vi "FindSimETH_CAn.vi"(6 "COM":string, 8 "error in":errorcluster) -> (0 "error out":errorcluster, 1 "Pass":bool, 2 "CmdOut":string)   [LabVIEW 2013]
panel:
  out "连接的字符串":string
  out "x >= 0?":bool
  out "数组":string[][](array[string])
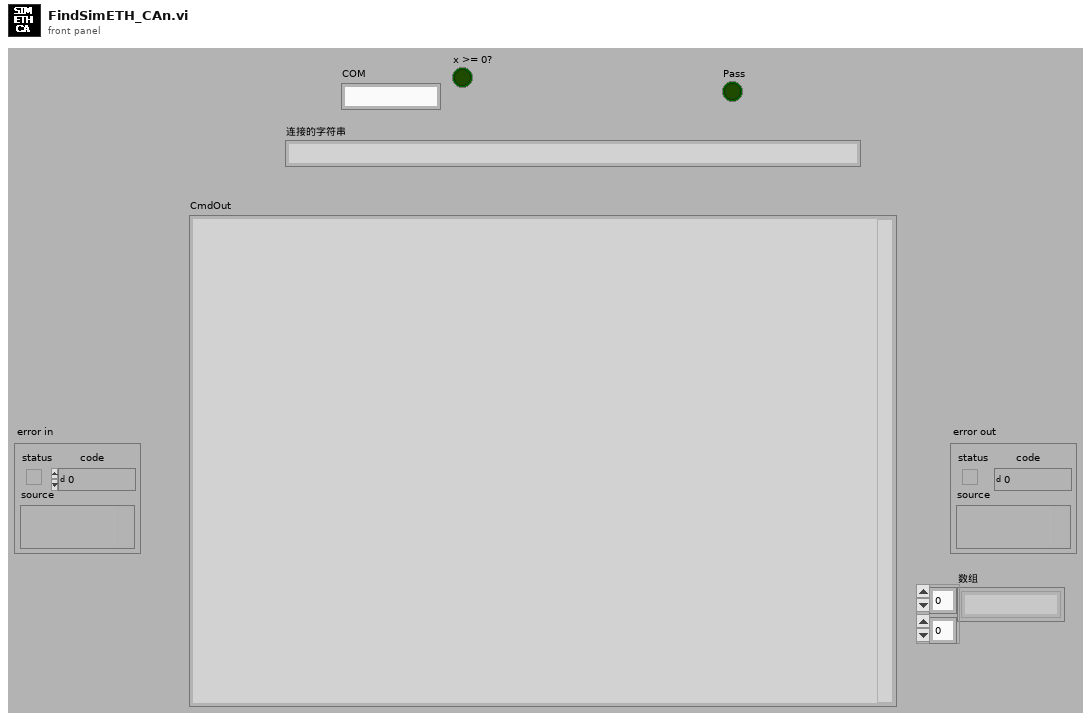
[diagram p1: front panel]
types:
  T1 = enum32{"invalid app kind", "Development System", "Run Time System", "Student Edition", "Embedded LabVIEW", "Evaluation", "Custom"}
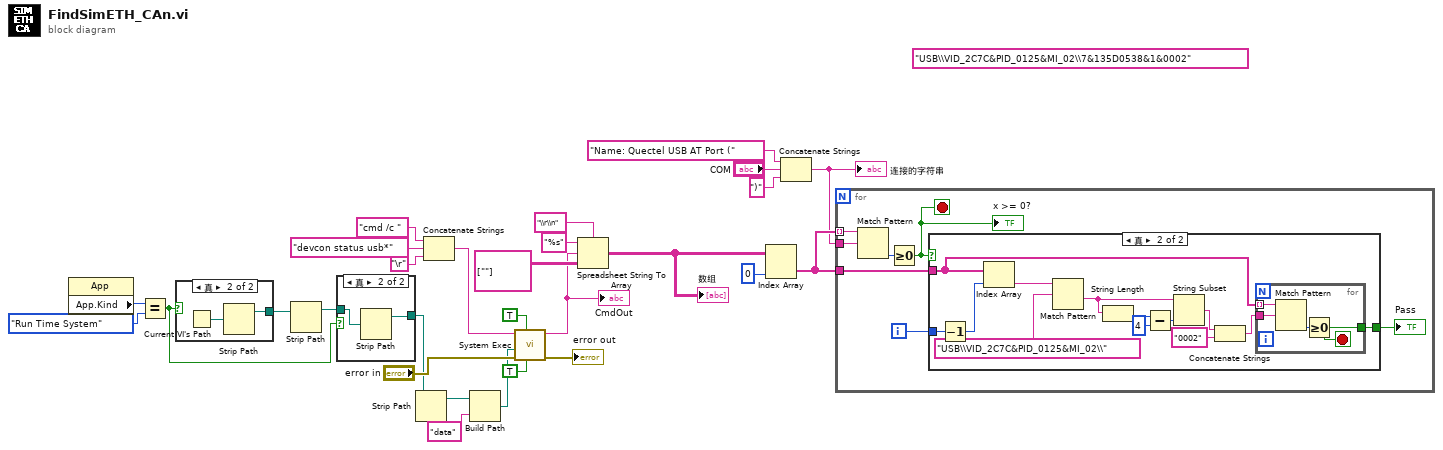
[diagram p0: block diagram]
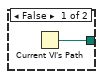
[diagram p3: hidden frame]
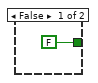
[diagram p4: hidden frame]
diagram:
  (unwired) "USB\\VID_2C7C&PID_0125&MI_02\\7&135D0538&1&0002" ("字符串")
  n1 = property class="App"() -> ("App.Kind"=w15:T1)  [unwired: 2 in, 2 out]
  n2 = Equal?(x=w15, y=T1."Run Time System") -> (x = y?=w5:bool)
  n3 = case shown="真" w5 {
    tunnel: [w29 w31] -> w14
    frame False {
      n4 = Current VI's Path() -> (path=w29:path)
    }
    frame True {
      n5 = Current VI's Path() -> (path=w30:path)
      n6 = Strip Path(path=w30) -> (stripped path=w31:path)  [unwired: 1 out]
    }
  }
  n7 = Strip Path(path=w14) -> (stripped path=w6:path)  [unwired: 1 out]
  n8 = case shown="真" w5 {
    tunnel: w6 -> [w32 w34]
    tunnel: [w32 w33] -> w4
    frame False {
    }
    frame True {
      n9 = Strip Path(path=w34) -> (stripped path=w33:path)  [unwired: 1 out]
    }
  }
  n10 = Strip Path(path=w4) -> (stripped path=w3:path)  [unwired: 1 out]
  n11 = Concatenate Strings("cmd /c " ("command line"), "devcon status usb*" ("command"), "\r") -> (w26:string)
  n12 = Build Path(base path=w3, name or relative path="data" ("名称或相对路径")) -> (appended path=w1:path)
  n13 = call <vilib>:"System Exec.vi"("run minimized? (F)"=TRUE, "wait until completion? (T)"=TRUE, "error in (no error)"="error in", "working directory"=w1, "command line"=w26) -> ("error out"=→"error out":errorcluster, "standard output"=w17:string)  [unwired: 1 in, 4 out]
  "CmdOut" <- w17
  n14 = Spreadsheet String To Array(delimiter (Tab)="\\r\\n" ("格式字符串"), format string="%s" ("格式字符串"), spreadsheet string=w17, array type (2D Dbl)=string[][] [[""]]) -> (array=w19:string[][])
  "数组" <- w19
  n15 = Index Array(array=w19, index (col)=0 ("索引 (行)")) -> (element=w11:string[])  [unwired: 1 in]
  n16 = Concatenate Strings("Name: Quectel USB AT Port (" ("command line"), "COM", ")" ("字符串")) -> (w8:string)
  "连接的字符串" <- w8
  n17 = for {
    tunnel: w11 -> [w41] mode=indexing
    tunnel: w8 -> [w40]
    tunnel: w11 -> [w38]
    i -> [w39]
    stop <- w36 stop-if-true
    n18 = Match Pattern(string=w41, regular expression=w40) -> (offset past match=w37:i32)  [unwired: 4 out]
    n19 = Greater Or Equal To 0?(x=w37) -> (x >= 0?=w36:bool)
    "x >= 0?" <- w36
    n20 = case shown="真" w36 {
      tunnel: w39 -> [_ w55]
      tunnel: w38 -> [_ w45]
      tunnel: [FALSE w43] -> w35
      frame False {
      }
      frame True {
        n21 = Decrement(x=w55) -> (x-1=w54:i32)
        n22 = Index Array(array=w45, index=w54) -> (element=w48:string)
        n23 = Match Pattern(string=w48, regular expression="USB\\VID_2C7C&PID_0125&MI_02\\" ("正则表达式")) -> (after substring=w52:string)  [unwired: 1 in, 3 out]
        n24 = String Length(string=w52) -> (length=w51:i32)
        n25 = Subtract(x=w51, y=4) -> (x-y=w49:i32)
        n26 = String Subset(string=w52, length (rest)=w49) -> (substring=w46:string)  [unwired: 1 in]
        n27 = Concatenate Strings(w46, "0002" ("字符串")) -> (w44:string)
        n28 = for {
          tunnel: w45 -> [w59] mode=indexing
          tunnel: [w57] -> w43
          tunnel: w44 -> [w56]
          stop <- w57 stop-if-true
          n29 = Match Pattern(string=w59, regular expression=w56) -> (offset past match=w58:i32)  [unwired: 1 in, 3 out]
          n30 = Greater Or Equal To 0?(x=w58) -> (x >= 0?=w57:bool)
        }
      }
    }
    "Pass" <- w35
  }
